vi "Case Structure Numeric.vi"() -> ()   [LabVIEW 2014]
panel:
  out "LED 3":bool
  out "LED 2":bool
  in  "Selector":u8(slide) scale=0.0..3.0
  in  "stop":bool
  out "LED 1":bool
  # "Using Case Structure"
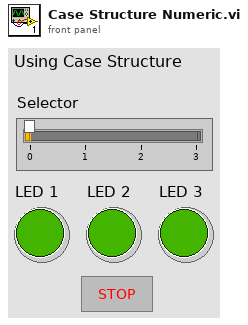
[diagram p1: front panel]
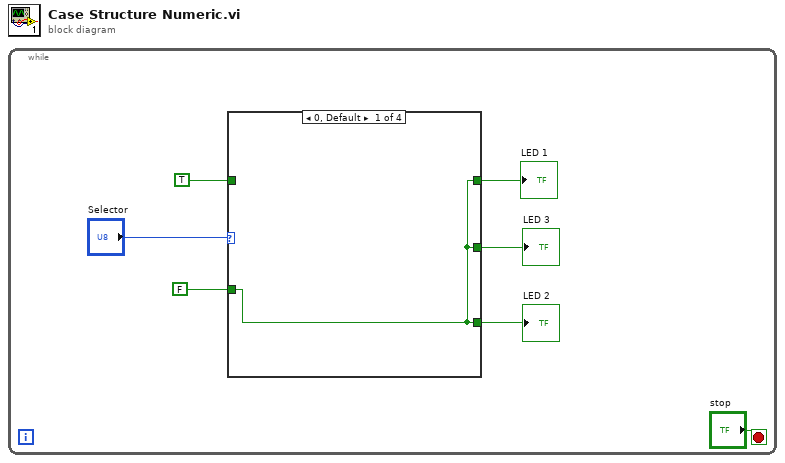
[diagram p0: block diagram]
diagram:
  n1 = while {
    stop <- "stop" stop-if-true
    n2 = case shown="0, Default" "Selector" {
      tunnel: [w8 w10 w11 w13] -> w6
      tunnel: TRUE -> [_ w10 w12 w14]
      tunnel: [w8 w9 w11 w14] -> w3
      tunnel: FALSE -> [w8 w9 w11 w13]
      tunnel: [w8 w9 w12 w13] -> w2
      frame 0, Default {
      }
      frame 1 {
      }
      frame 2 {
      }
      frame 3 {
      }
    }
    "LED 1" <- w6
    "LED 3" <- w3
    "LED 2" <- w2
  }
